vi "scaling.vi"(5 "x":sgl[](array[numeric]), 6 "Offset":sgl, 8 "raw max":sgl, 9 "raw min":sgl, 10 "emin":sgl, 11 "emax":sgl) -> (2 "Y":sgl[](array[numeric]))   [LabVIEW 2018]
panel:
  out "error out":errorcluster
  in  "error in (no error)":errorcluster
  out "c":sgl
  out "m":sgl
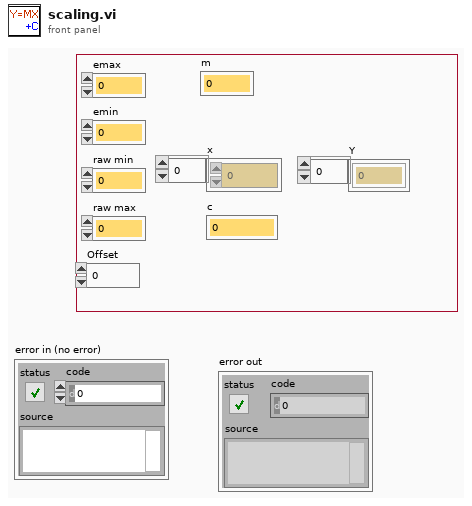
[diagram p1: front panel]
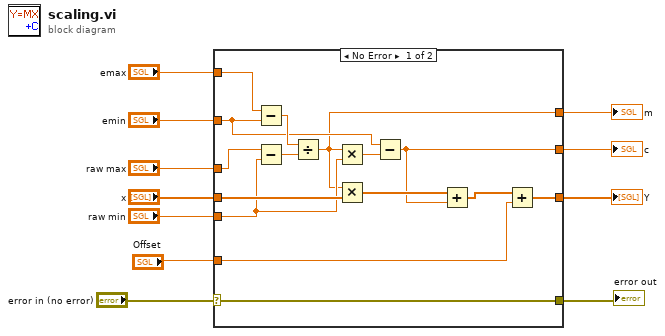
[diagram p0: block diagram]
diagram:
  n1 = case shown="No Error" "error in (no error)" {
    selector: "error in (no error)" -> [w20 w27]
    tunnel: "emin" -> [w19 _]
    tunnel: "raw min" -> [w18 _]
    tunnel: "x" -> [w24 _]
    tunnel: "emax" -> [w17 _]
    tunnel: "raw max" -> [w15 _]
    tunnel: [w16 _] -> w6
    tunnel: [w14 _] -> w5
    tunnel: [w21 _] -> w4
    tunnel: [w20 w27] -> w2
    tunnel: "Offset" -> [w12 _]
    frame No Error {
      n2 = Subtract(x=w17, y=w19) -> (x-y=w26:sgl)
      n3 = Subtract(x=w15, y=w18) -> (x-y=w25:sgl)
      n4 = Divide(x=w26, y=w25) -> (x/y=w16:sgl)
      n5 = Multiply(x=w16, y=w18) -> (x*y=w23:sgl)
      n6 = Multiply(x=w16, y=w24) -> (x*y=w22:sgl[])
      n7 = Subtract(x=w19, y=w23) -> (x-y=w21:sgl)
      n8 = Add(x=w22, y=w21) -> (x+y=w13:sgl[])
      n9 = Add(x=w13, y=w12) -> (x+y=w14:sgl[])
    }
    frame Error {
    }
  }
  "error out" <- w2
  "m" <- w6
  "Y" <- w5
  "c" <- w4
